vi "F8588A set & read using driver.vi"() -> ()   [LabVIEW 2020]
uses:
  F8588A Coupling.ctl
panel:
  out "Waveform Graph":dbl[](graph)
  out "error out":errorcluster
  out "waveform data [V]":dbl[](array[numeric])
  out "read samples":i32
  in  "samples count (100)":i32=100
  out "idn string":string
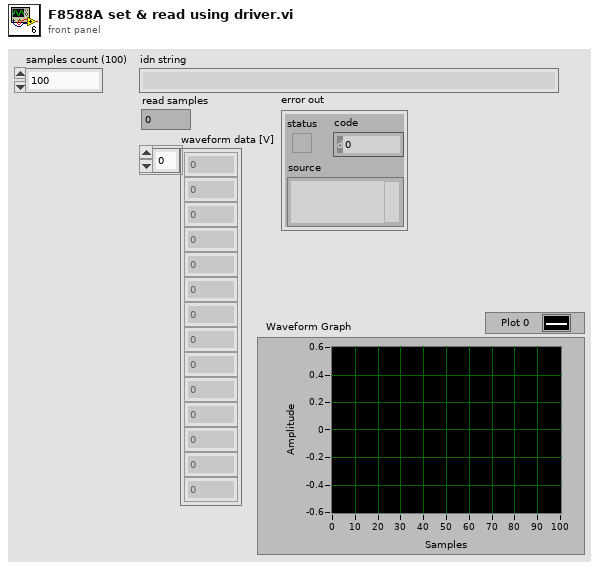
[diagram p1: front panel]
types:
  T1 = typedef "F8588A Coupling.ctl" = enum16{"AC, 1 MOhm", "AC, 10 MOhm", "DC, 1 MOhm", "DC, 10 MOhm", "DC, auto"}
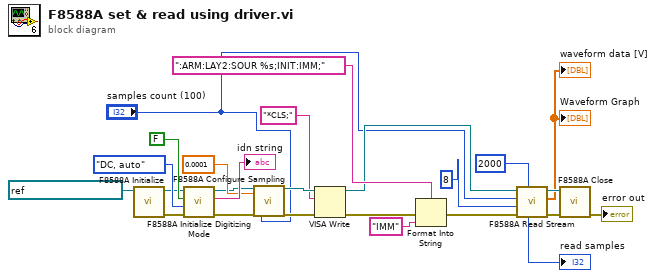
[diagram p0: block diagram]
diagram:
  n1 = call "F8588A Initialize.vi"("VISA resource name"=refnum<visa-resource-name> "GPIB0::10::INSTR") -> ("error out"=w24:errorcluster, "VISA resource name out"=w12:refnum<visa-resource-name>)  [unwired: 8 in, 1 out]
  n2 = call "F8588A Initialize Digitizing Mode.vi"("error in (no error)"=w24, "dmm couple (DC auto)"=F8588A_Coupling."DC, auto", "Reset (True)"=FALSE, "VISA DMM"=w12) -> ("error out"=w25:errorcluster, "idn string"=→"idn string":string, "VISA resource name out"=w13:refnum<visa-resource-name>)  [unwired: 4 in, 1 out]
  n3 = call "F8588A Configure Sampling.vi"("VISA resource in"=w13, "sample period [s] (-1: use EXT trig as source)"=0.0001, "error in"=w25, "samples count (100)"="samples count (100)") -> ("VISA resource name out"=w15:refnum<visa-resource-name>, "error out"=w18:errorcluster)  [unwired: 14 in]
  n4 = VISA Write(VISA resource name=w15, write buffer="*CLS;", error in (no error)=w18) -> (VISA resource name out=w10:refnum<visa-resource-name>, error out=w17:errorcluster)  [unwired: 1 out]
  n5 = Format Into String(format string=":ARM:LAY2:SOUR %s;INIT:IMM;" ("write buffer"), error in=w17, "IMM" ("initial string")) -> (error out=w2:errorcluster)  [unwired: 1 in, 1 out]
  n6 = call "F8588A Read Stream.vi"("read timeout [ms] (30000s)"=u32 2000, "error in (no error)"=w2, "sample size [B]"=8, "samples count"="samples count (100)", "VISA session"=w10) -> ("error out"=w23:errorcluster, "waveform data [V]"=→"waveform data [V]" →"Waveform Graph":dbl[], "dup VISA session"=w8:refnum<visa-resource-name>, "read samples"=→"read samples":i32)  [unwired: 1 in, 2 out]
  n7 = call "F8588A Close.vi"("error in (no error)"=w23, "VISA resource name"=w8) -> ("error out"=→"error out":errorcluster)  [unwired: 9 in]
